vi "Simulate iRobot Open.vi"(10 "step size (mSec)":u32=2 min=1, 11 "enable 3D visualization (T)":bool=TRUE) -> (0 "error out":errorcluster, 2 "initial position":sgl[](array[numeric]), 3 "Cal Climber":T1)   [LabVIEW 2013]
doc: "Begins a simulation of the Cal Climber."
uses:
  Simulate iRobot.ctl
  <instrlib>/DC Motor Controller/HAIOL/DC Motor Controller.lvclass
  <vilib>/robotics/Simulator/Engine/ctl/DeviceID.ctl
  <vilib>/robotics/Simulator/Interface/Simulator References/Get Robot Body Reference.vi
  <vilib>/robotics/Simulator/Interface/Simulator References/Get Sensor Reference.vi
  <vilib>/robotics/Simulator/NI_Robotics_Simulator.lvlib
  <resource>/objmgr/LVODE.rc
  <instrlib>/DC Motor Controller/HAIOL/Simulator/DC Motor Controller Simulator.lvclass
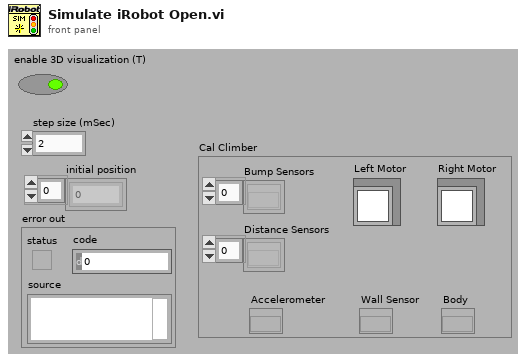
[diagram p1: front panel]
types:
  T1 = typedef "Simulate iRobot.ctl" = cluster{"Bump Sensors":refnum<k20>[], "Distance Sensors":refnum<k20>[], "Accelerometer":refnum<k20>, "Wall Sensor":refnum<k20>, "Body":refnum<k20>, "Left Motor":refnum<class "DC Motor Controller.lvclass">, "Right Motor":refnum<class "DC Motor Controller.lvclass">}
  T2 = typedef "NI_Robotics_Simulator.lvlib/DeviceID.ctl" = cluster{"robot ID":string, "sensor/actuator ID":string}
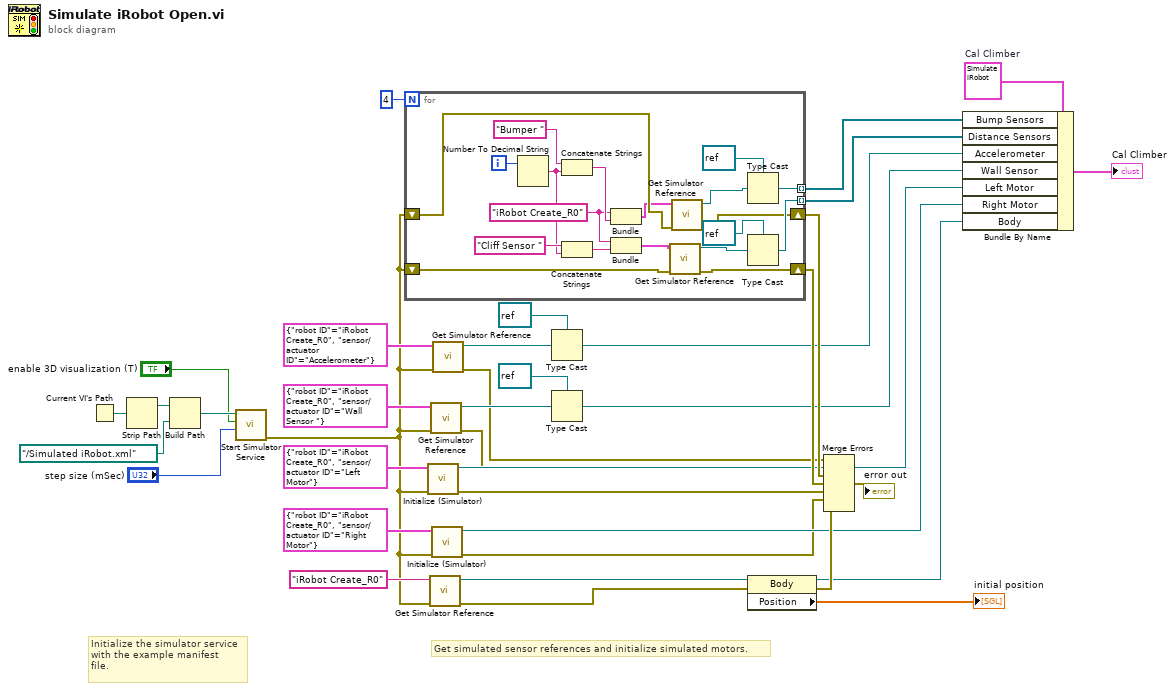
[diagram p0: block diagram]
diagram:
  w28 = T1 {"Bump Sensors"=[], "Distance Sensors"=[], "Accelerometer"=refnum, "Wall Sensor"=refnum, "Body"=refnum, "Left Motor"=refnum, "Right Motor"=refnum}  # Cal Climber
  # "Get simulated sensor references and initialize simulated motors."
  # "Initialize the simulator service\nwith the example manifest\nfile."
  n1 = Current VI's Path() -> (path=w2:path)
  n2 = Strip Path(path=w2) -> (stripped path=w37:path)  [unwired: 1 out]
  n3 = Build Path(base path=w37, name or relative path=path "../Simulated iRobot.xml" ("Simulation Manifest File")) -> (appended path=w3:path)
  n4 = call <vilib>:"Start Simulator Service.vi"("step size (ms)"="step size (mSec)", "enable 3D visualization (T)"="enable 3D visualization (T)", "manifest file"=w3) -> ("error out"=w9:errorcluster)  [unwired: 8 in]
  n5 = for {
    N: 4 -> [_]
    tunnel: [w53] -> w29 mode=indexing
    tunnel: [w47] -> w30 mode=indexing
    shift-right: [w42] -> w32
    shift-left: w9 -> [w45]
    shift-right: [w39] -> w33
    shift-left: w9 -> [w40]
    i -> [w56]
    w46 = "iRobot Create_R0" ("Robot ID")
    n6 = Number To Decimal String(number=w56) -> (decimal integer string=w50:string)  [unwired: 1 in]
    n7 = Concatenate Strings("Bumper " ("Device Label"), w50) -> (w49:string)
    n8 = Concatenate Strings("Cliff Sensor " ("Device Label"), w50) -> (w54:string)
    n9 = Bundle("Robot ID"=w46, w49) -> (w44:cluster{"Robot ID":string, string})  [unwired: 1 in]
    n10 = Bundle("Robot ID"=w46, w54) -> (w41:cluster{"Robot ID":string, string})  [unwired: 1 in]
    n11 = call-poly <vilib>:"Get Simulator Reference.vi"("error in (no error)"=w40, "device ID"=w41) -> ("error out"=w39:errorcluster, "sensor ref"=w38:refnum<k20>)  [unwired: 8 in]
    n12 = call-poly <vilib>:"Get Simulator Reference.vi"("error in (no error)"=w45, "device ID"=w44) -> ("error out"=w42:errorcluster, "sensor ref"=w43:refnum<k20>)  [unwired: 8 in]
    n13 = Type Cast(type=refnum<k20> refnum ("DistanceSensor Out"), x=w43) -> (*(type *) &x=w47:refnum<k20>)
    n14 = Type Cast(type=refnum<k20> refnum ("DistanceSensor Out"), x=w38) -> (*(type *) &x=w53:refnum<k20>)
  }
  n15 = call <instrlib>:"Initialize (Simulator).vi"("error in (no error)"=w9, "Device ID"=T2 {"robot ID"="iRobot Create_R0", "sensor/actuator ID"="Left Motor"}) -> ("error out"=w14:errorcluster, "DC Motor Controller out"=w15:refnum<class "DC Motor Controller.lvclass">)  [unwired: 8 in]
  n16 = call-poly <vilib>:"Get Simulator Reference.vi"("error in (no error)"=w9, "robot ID"="iRobot Create_R0" ("Robot ID")) -> ("error out"=w7:errorcluster, "robot body ref"=w8:refnum<k20>)  [unwired: 8 in]
  n17 = call-poly <vilib>:"Get Simulator Reference.vi"("error in (no error)"=w9, "device ID"=T2 {"robot ID"="iRobot Create_R0", "sensor/actuator ID"="Wall Sensor "} ("Device ID")) -> ("error out"=w6:errorcluster, "sensor ref"=w17:refnum<k20>)  [unwired: 8 in]
  n18 = call <instrlib>:"Initialize (Simulator).vi"("error in (no error)"=w9, "Device ID"=T2 {"robot ID"="iRobot Create_R0", "sensor/actuator ID"="Right Motor"}) -> ("error out"=w11:errorcluster, "DC Motor Controller out"=w12:refnum<class "DC Motor Controller.lvclass">)  [unwired: 8 in]
  n19 = call-poly <vilib>:"Get Simulator Reference.vi"("error in (no error)"=w9, "device ID"=T2 {"robot ID"="iRobot Create_R0", "sensor/actuator ID"="Accelerometer"} ("Device ID")) -> ("error out"=w5:errorcluster, "sensor ref"=w19:refnum<k20>)  [unwired: 8 in]
  n20 = Type Cast(type=refnum<k20> refnum ("DistanceSensor Out"), x=w19) -> (*(type *) &x=w27:refnum<k20>)
  n21 = Type Cast(type=refnum<k20> refnum ("DistanceSensor Out"), x=w17) -> (*(type *) &x=w26:refnum<k20>)
  n22 = property class="Body"(reference=w8, error in=w7) -> (reference out=w25:refnum<k20>, error out=w31:errorcluster, "Position"=→"initial position":sgl[])
  n23 = Merge Errors(w5, w6, w32, w33, w14, w11, w31) -> (→"error out":errorcluster)
  n24 = Bundle By Name(cluster=w28, "Bump Sensors"=w30, "Distance Sensors"=w29, "Accelerometer"=w27, "Wall Sensor"=w26, "Left Motor"=w15, "Right Motor"=w12, "Body"=w25) -> (→"Cal Climber":T1)
